vi "InsertData.vi"(8 "error in (no error)":errorcluster, 10 "Data Cluster":variant, 11 "object in":refnum<class "TableLogger_CSV_Actor.lvclass">) -> (0 "error out":errorcluster, 3 "object out":refnum<class "TableLogger_CSV_Actor.lvclass">)   [LabVIEW 2014, in "TableLogger_CSV_Actor.lvlib" / "TableLogger_CSV_Actor.lvclass"]
uses:
  TableLogger_CSV_Actor.lvclass
  TableLogger_CSV_Actor.lvclass/TableLogger_CSV_Actor.ctl
  TableLogger_Actor/TableLogger_Actor/TableLogger_Actor.lvclass
panel:
  # "Connector Pane"
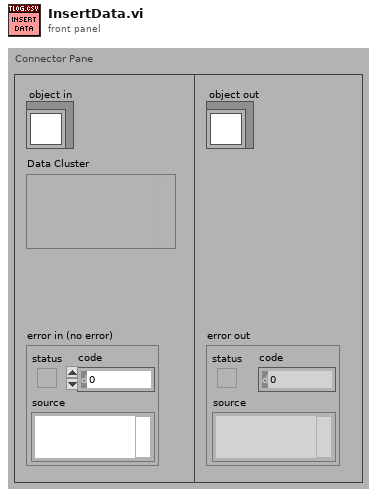
[diagram p1: front panel]
types:
  T1 = typedef "Type Descriptor Enumeration__ogtk.ctl" = enum8{"<Null>", "I8", "I16", "I32", "I64", "U8", "U16", "U32", "U64", "SGL", "DBL", "EXT", "CSG", "CDB", "CXT", "0x0F", "0x10", "0x11", "0x12", "0x13", "0x14", "Enum U8", "Enum U16", "Enum U32", "Enum U64", "SGL PQ", "DBL PQ", "EXT PQ", "CSG PQ", "CDB PQ", "CXT PQ", "0x1F", "0x20", "Boolean", "0x22", "0x23", "0x24", "0x25", "0x26", "0x27", "0x28", "0x29", "0x2A", "0x2B", "0x2C", "0x2D", "0x2E", "0x2F", "String", "0x31", "Path", "Pict", "0x34", "0x35", "0x36", "DAQ", "0x38", "0x39", "0x3A", "0x3B", "0x3C", "0x3D", "0x3E", "0x3F", "Array", "0x41", "0x42", "0x43", "0x44", "0x45", "0x46", "0x47", "0x48", "0x49", "0x4A", "0x4B", "0x4C", "0x4D", "0x4E", "0x4F", "Cluster", "0x51", "0x52", "Variant", "Waveform", "0x55", "0x56", "0x57", "0x58", "0x59", "0x5A", "0x5B", "0x5C", "0x5D", "0x5E", "0x5F", "0x60", "0x61", "0x62", "0x63", "0x64", "0x65", "0x66", "0x67", "0x68", "0x69", "0x6A", "0x6B", "0x6C", "0x6D", "0x6E", "0x6F", "Refnum"}
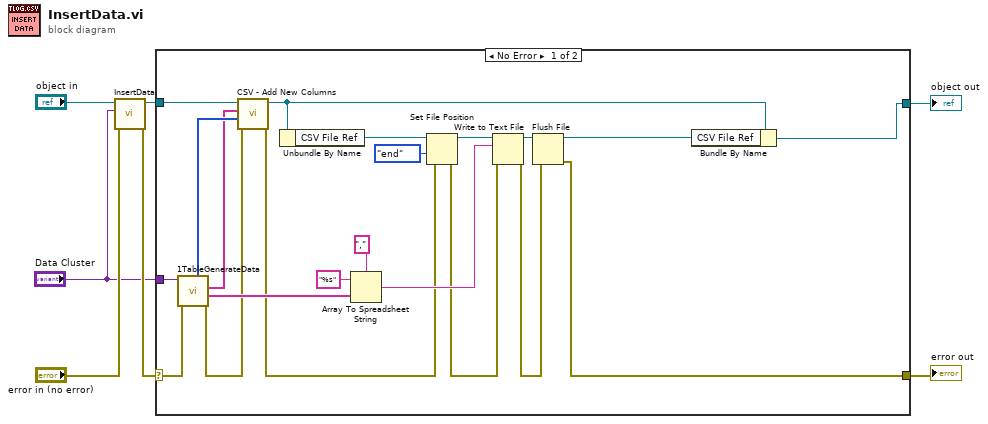
[diagram p0: block diagram]
diagram:
  n1 = call-parent "InsertData.vi"("error in (no error)"="error in (no error)", "Data Cluster"="Data Cluster", "object in"="object in") -> ("error out"=w2:errorcluster, "object out"=w4:refnum<class "TableLogger_CSV_Actor.lvclass">)  [unwired: 7 in]
  n2 = case shown="No Error" w2 {
    selector: w2 -> [w27 w30]
    tunnel: [w8 w30] -> w7
    tunnel: [w11 w29] -> w6
    tunnel: w4 -> [w22 w29]
    tunnel: "Data Cluster" -> [w28 _]
    frame No Error {
      n3 = call "1TableGenerateData.vi"("error in (no error)"=w27, "Cluster Variant"=w28) -> ("error out"=w20:errorcluster, "Data"=w23:string[], "Headers"=w9:string[], "LV Data Types"=w10:T1[])  [unwired: 5 in, 1 out]
      n4 = call "CSV - Add New Columns.vi"("error in (no error)"=w20, "LV Data Types"=w10, "Headers"=w9, "TableLogger_CSV_Actor in"=w22) -> ("error out"=w18:errorcluster, "TableLogger_CSV_Actor out"=w21:refnum<class "TableLogger_CSV_Actor.lvclass">)  [unwired: 6 in]
      n5 = Unbundle By Name(w21) -> ("CSV File Ref"=w16:refnum<file>)
      n6 = Array To Spreadsheet String(delimiter (Tab)=",", array=w23, 3:"%s" ("format string")) -> (spreadsheet string=w26:string)
      n7 = Set File Position(refnum=w16, from (0:start)=enum16{"start", "end", "current"}."end", error in=w18) -> (refnum out=w15:refnum<file>, error out=w17:errorcluster)  [unwired: 1 in]
      n8 = Write to Text File(file (use dialog)=w15, text=w26, error in=w17) -> (refnum out=w14:refnum<file>, error out=w13:errorcluster)  [unwired: 1 in, 1 out]
      n9 = Flush File(refnum=w14, error in=w13) -> (refnum out=w12:refnum<file>, error out=w8:errorcluster)
      n10 = Bundle By Name(cluster=w21, "CSV File Ref"=w12) -> (w11:refnum<class "TableLogger_CSV_Actor.lvclass">)
    }
    frame Error {
    }
  }
  "error out" <- w7
  "object out" <- w6
